vi "LESO_queue_status.vi"(7 "milliseconds to wait":u32, 8 "error in":errorcluster, 11 "Handle in":u32) -> (0 "error out":errorcluster, 1 "Bytes Waiting":u32, 2 "FT_Status":u32(ring) items=["FT_OK", "FT_INVALID_HANDLE", "FT_DEVICE_NOT_FOUND", "FT_DEVICE_NOT_OPENED", "FT_IO_ERROR", "FT_INSUFFICIENT_RESOURCES", "FT_INVALID_PARAMETER", "FT_INVALID_BAUD_RATE", "FT_DEVICE_NOT_OPENED_FOR_ERASE", "FT_DEVICE_NOT_OPENED_FOR_WRITE", "FT_FAILED_TO_WRITE_DEVICE", "FT_EEPROM_READ_FAILED", "FT_EEPROM_WRITE_FAILED", "FT_EEPROM_ERASE_FAILED", "FT_EEPROM_NOT_PRESENT", "FT_EEPROM_NOT_PROGRAMMED", "FT_INVALID_ARGS", "FT_NOT_SUPPORTED", "FT_OTHER_ERROR"], 3 "Handle out":u32)   [LabVIEW 2012]
doc: "Возвращает число байт в очереди приема доступных для чтения."
uses:
  FTD2XX.dll
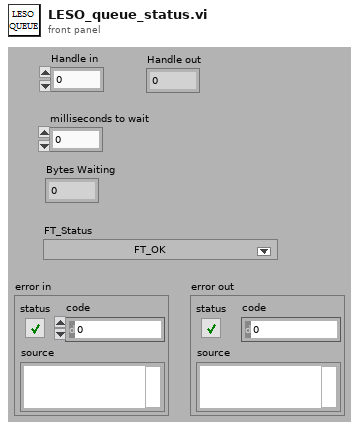
[diagram p1: front panel]
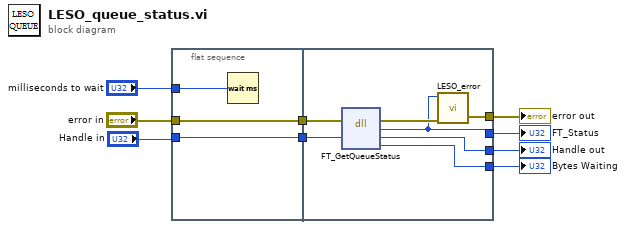
[diagram p0: block diagram]
diagram:
  n1 = flat-sequence {
    tunnel: "Handle in" -> [w12]
    tunnel: [w12] -> w7
    tunnel: "error in" -> [w11]
    tunnel: [w11] -> w6
    tunnel: "milliseconds to wait" -> [w10]
    tunnel: [w15] -> w9
    tunnel: [w19] -> w8
    tunnel: w7 -> [w18]
    tunnel: w6 -> [w17]
    tunnel: [w14] -> w1
    tunnel: [w13] -> w3
    frame #0 {
      n2 = Wait (ms)(milliseconds to wait=w10) -> ()  [unwired: 1 out]
    }
    frame #1 {
      n3 = dll-call lib="FTD2XX.dll" fn="FT_GetQueueStatus"(error in=w17, "Handle"=w18) -> (error out=w16:errorcluster, "FT_Status"=w15:u32, "Handle"=w13:u32, "BytesWaiting"=w19:u32)  [unwired: 3 in, 1 out]
      n4 = call "LESO_error.vi"("error in"=w16, "FT_Status"=w15) -> ("error out"=w14:errorcluster)  [unwired: 9 in]
    }
  }
  "FT_Status" <- w9
  "Bytes Waiting" <- w8
  "Handle out" <- w3
  "error out" <- w1
